vi "SetPiplelineImageBuffer.vi"(8 "error in (no error)":errorcluster, 10 "ImageBuffers":refnum<queue>, 11 "Microscope in":refnum<class "Microscope.lvclass">) -> (0 "error out":errorcluster, 3 "Microscope out":refnum<class "Microscope.lvclass">)   [LabVIEW 2020, in "Microscope.lvlib" / "Microscope.lvclass"]
uses:
  Microscope.lvclass
  <vilib>/vision/Image Controls.llb/IMAQ Image.ctl
  Microscope.lvclass/Microscope.ctl
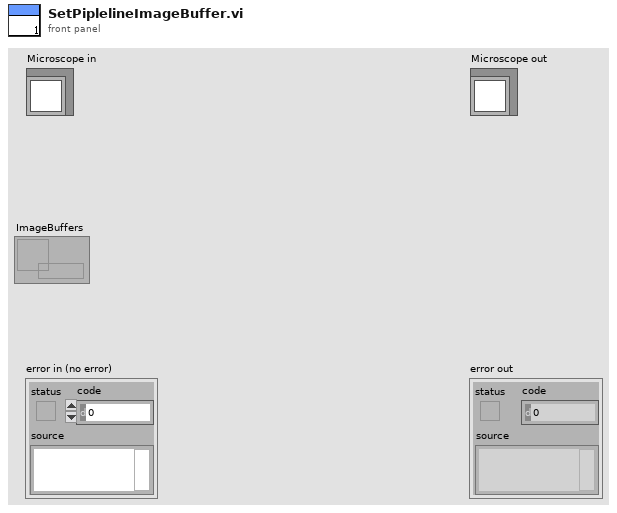
[diagram p1: front panel]
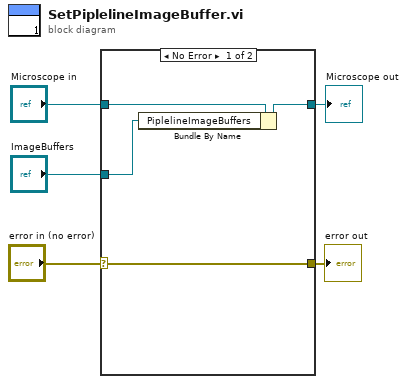
[diagram p0: block diagram]
diagram:
  n1 = case shown="No Error" "error in (no error)" {
    selector: "error in (no error)" -> [w6 w11]
    tunnel: [w6 w11] -> w4
    tunnel: "Microscope in" -> [w9 w10]
    tunnel: [w8 w10] -> w2
    tunnel: "ImageBuffers" -> [w7 _]
    frame No Error {
      n2 = Bundle By Name(cluster=w9, "PiplelineImageBuffers"=w7) -> (w8:refnum<class "Microscope.lvclass">)
    }
    frame Error {
    }
  }
  "error out" <- w4
  "Microscope out" <- w2
